vi "Initialize FPGA (iSUB) (SubVI).vi"(7 "Image Size":T2={"Height"=2048, "Width"=2048}, 11 "FPGA REF (iSUB) IN":T1) -> (0 "Camera OK?":bool, 3 "FPGA REF (iSUB) OUT":T1)   [LabVIEW 2015]
uses:
  Controls (HOST)/Image Size.ctl
  Controls (HOST)/FPGA REF (iSUB).ctl
  <vilib>/rvi/interface/common/niFpgaWaitOnOcc.vi
  <vilib>/Utility/error.llb/Error Cluster From Error Code.vi
  <vilib>/rvi/errors/niLvFpgaAdjustHostInterfaceError.vi
  <vilib>/FPGAPlugInAG/Dynamic/niLvFpga_Run_Dynamic.vi
  <vilib>/rvi/interface/nirviMethod/nirviMethod.xnode
  <vilib>/rvi/interface/nirviReadWriteControl/nirviReadWriteControl.xnode
  <vilib>/rvi/errors/niLvFpgaMergeErrorWithErrorCode.vi
  <vilib>/rvi/interface/Simulation/niFpgaSimulationCallBeginRW.vi
  <vilib>/FPGAPlugInAG/Dynamic/niLvFpga_ConfigureFifo_Dynamic.vi
  <vilib>/FPGAPlugInAG/Dynamic/niLvFpga_StartFifo_Dynamic.vi
  NiFpgaLv.dll
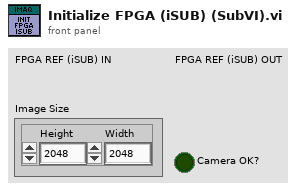
[diagram p1: front panel]
types:
  T1 = typedef "FPGA REF (iSUB).ctl" = refnum<k20>
  T2 = typedef "Image Size.ctl" = cluster{"Height":u16, "Width":u16}
  T3 = enum8{"Standard", "Basler 10-tap", "Vosskühler 10-tap"}
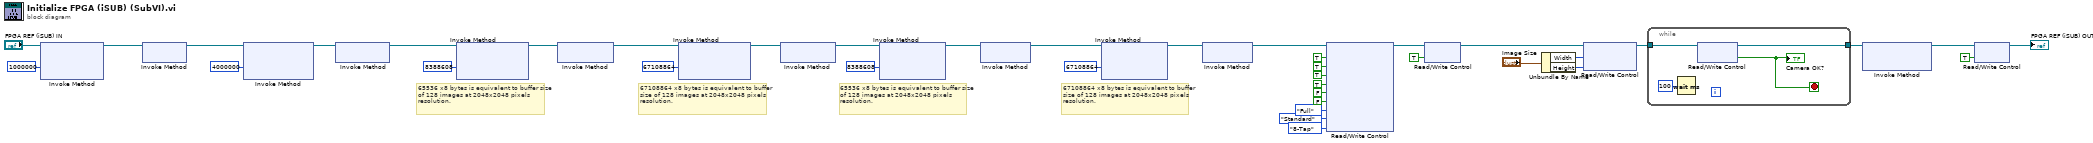
[diagram p0: block diagram]
diagram:
  # "65536 x8 bytes is equivalent to buffer size of 128 images at 2048x2048 pixels resolution."
  # "67108864 x8 bytes is equivalent to buffer size of 128 images at 2048x2048 pixels resolution."
  # "65536 x8 bytes is equivalent to buffer size of 128 images at 2048x2048 pixels resolution."
  # "67108864 x8 bytes is equivalent to buffer size of 128 images at 2048x2048 pixels resolution."
  n1 = xnode "Invoke Method"("FPGA VI Reference In"="FPGA REF (iSUB) IN", "Requested Depth"=u32 1000000) -> ("FPGA VI Reference Out"=w21:T1)  [unwired: 1 in, 2 out]
  n2 = xnode "Invoke Method"("FPGA VI Reference In"=w21) -> ("FPGA VI Reference Out"=w10:T1)  [unwired: 1 in, 1 out]
  n3 = xnode "Invoke Method"("FPGA VI Reference In"=w10, "Requested Depth"=u32 4000000) -> ("FPGA VI Reference Out"=w11:T1)  [unwired: 1 in, 2 out]
  n4 = xnode "Invoke Method"("FPGA VI Reference In"=w11) -> ("FPGA VI Reference Out"=w2:T1)  [unwired: 1 in, 1 out]
  n5 = xnode "Invoke Method"("FPGA VI Reference In"=w2, "Requested Depth"=u32 8388608) -> ("FPGA VI Reference Out"=w6:T1)  [unwired: 1 in, 2 out]
  n6 = xnode "Invoke Method"("FPGA VI Reference In"=w6) -> ("FPGA VI Reference Out"=w7:T1)  [unwired: 1 in, 1 out]
  n7 = xnode "Invoke Method"("FPGA VI Reference In"=w7, "Requested Depth"=u32 67108864) -> ("FPGA VI Reference Out"=w3:T1)  [unwired: 1 in, 2 out]
  n8 = xnode "Invoke Method"("FPGA VI Reference In"=w3) -> ("FPGA VI Reference Out"=w1:T1)  [unwired: 1 in, 1 out]
  n9 = xnode "Invoke Method"("FPGA VI Reference In"=w1, "Requested Depth"=u32 8388608) -> ("FPGA VI Reference Out"=w19:T1)  [unwired: 1 in, 2 out]
  n10 = xnode "Invoke Method"("FPGA VI Reference In"=w19) -> ("FPGA VI Reference Out"=w18:T1)  [unwired: 1 in, 1 out]
  n11 = xnode "Invoke Method"("FPGA VI Reference In"=w18, "Requested Depth"=u32 67108864) -> ("FPGA VI Reference Out"=w29:T1)  [unwired: 1 in, 2 out]
  n12 = xnode "Invoke Method"("FPGA VI Reference In"=w29) -> ("FPGA VI Reference Out"=w39:T1)  [unwired: 1 in, 1 out]
  n13 = xnode "Read/Write Control"("FPGA VI Reference In"=w39, "FVAL Active High"=TRUE ("IO Module Config.CL FVAL Active High"), "LVAL Active High"=TRUE ("IO Module Config.CL LVAL Active High"), "DVAL Active High"=TRUE ("IO Module Config.CL DVAL Active High"), "Spare Active High"=TRUE ("IO Module Config.CL Spare Active High"), "Line Scan"=FALSE, "Ignore DVAL"=FALSE ("CL Config.Line Scan"), "Configuration"=enum8{"Base", "Medium", "Full"}."Full" ("CL Config.Configuration"), "Signal Mapping"=T3."Standard" ("CL Config.Signal Mapping"), "Tap Configuration"=enum8{"8-Tap", "10-Tap"}."8-Tap") -> ("FPGA VI Reference Out"=w17:T1)  [unwired: 1 in, 1 out]
  n14 = xnode "Read/Write Control"("FPGA VI Reference In"=w17, "Initialize"=TRUE ("Arm Acquisition")) -> ("FPGA VI Reference Out"=w26:T1)  [unwired: 1 in, 1 out]
  n15 = Unbundle By Name("Image Size") -> ("Width"=w14:u16, "Height"=w13:u16)
  n16 = xnode "Read/Write Control"("FPGA VI Reference In"=w26, "Image Width"=w14, "Image Height"=w13) -> ("FPGA VI Reference Out"=w16:T1)  [unwired: 1 in, 1 out]
  n17 = while {
    tunnel: w16 -> [w43]
    tunnel: [w42] -> w25
    stop <- w40 stop-if-true
    n18 = Wait (ms)(milliseconds to wait=u32 100) -> ()  [unwired: 1 out]
    n19 = xnode "Read/Write Control"("FPGA VI Reference In"=w43) -> ("FPGA VI Reference Out"=w42:T1, "Initialized"=w40:bool)  [unwired: 1 in, 1 out]
    "Camera OK?" <- w40
  }
  n20 = xnode "Invoke Method"("FPGA VI Reference In"=w25) -> ("FPGA VI Reference Out"=w24:T1)  [unwired: 2 in, 1 out]
  n21 = xnode "Read/Write Control"("FPGA VI Reference In"=w24, "Acquire"=TRUE ("Acq Control.Acquire")) -> ("FPGA VI Reference Out"=→"FPGA REF (iSUB) OUT":T1)  [unwired: 1 in, 1 out]
